vi "Add Database.vi"(8 "error in":errorcluster, 10 "Custom XML":string, 11 "Node Ptr":u64 format="%.0x") -> (0 "error out":errorcluster, 3 "Device Item Ref out":T1 format="%.0x")   [LabVIEW 2020, in "Communication Bus Template System Explorer.lvlib"]
uses:
  <vilib>/NI VeriStand/Custom Device API/Custom Device Item Ref.ctl
  Shared/Constants.vi
  Communication Bus Template System Explorer.lvlib
  <vilib>/NI VeriStand/Custom Device API/Custom Device API.lvlib
  Shared/Communication Bus Template Shared.lvlib
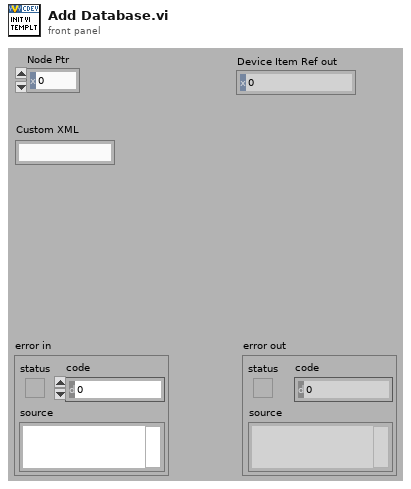
[diagram p1: front panel]
types:
  T1 = typedef "Custom Device API.lvlib/Custom Device Item Ref.ctl" = u64
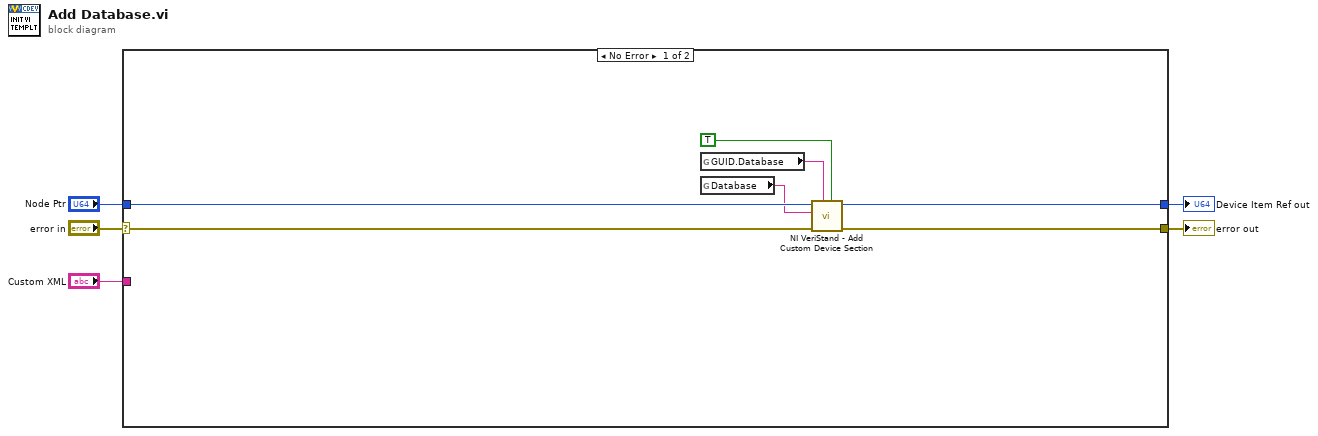
[diagram p0: block diagram]
diagram:
  n1 = case shown="No Error" "error in" {
    selector: "error in" -> [w11 w14]
    tunnel: [w10 w14] -> w5
    tunnel: [w9 w13] -> w3
    tunnel: "Node Ptr" -> [w12 w13]
    tunnel: "Custom XML" -> [_ _]
    frame No Error {
      n2 = global read "Constants.vi" "GUID.Database"() -> (w7:string)
      n3 = global read "Constants.vi" "Database"() -> (w8:string)
      n4 = call <vilib>:"NI VeriStand - Add Custom Device Section.vi"("Highlight? (F)"=TRUE, "GUID (Default Section)"=w7, "error in (no error)"=w11, "Section Name"=w8, "Parent Ref in"=w12) -> ("error out"=w10:errorcluster, "Parent Ref out"=w9:T1)  [unwired: 3 in, 2 out]
    }
    frame Error {
    }
  }
  "error out" <- w5
  "Device Item Ref out" <- w3
